vi "decay fit.vi"() -> ()   [LabVIEW 2015]
uses:
  <vilib>/Utility/file.llb/Read Delimited Spreadsheet (DBL).vi
panel:
  out "XY Graph":cluster{"all rows":dbl[], "all rows":dbl[]}[](graph)=[{"all rows"=[5.0, 6.0, 7.0, 8.0, 9.0, 10.0, 11.0, 12.0, 13.0, 14.0, 15.0, 16.0, 17.0, 18.0, 19.0, 20.0, 21.0, 22.0, 23.0, 24.0, 25.0, 26.0, 27.0, 28.0, 29.0, 30.0, 31.0, 32.0, 33.0, 34.0, 35.0, 36.0, 37.0, 38.0, 39.0, 40.0, 41.0, 42.0, 43.0, 44.0, 45.0, 46.0, 47.0, 48.0, 49.0, 50.0, 51.0, 52.0, 53.0, 54.0, 55.0, 56.0, 57.0, 58.0, 59.0, 60.0, 61.0, 62.0, 63.0, 64.0, 65.0, 66.0, 67.0, 68.0, 69.0, 70.0, 71.0, 72.0, 73.0, 74.0, 75.0, 76.0, 77.0, 78.0, 79.0, 80.0, 81.0, 82.0, 83.0, 84.0, 85.0, 86.0, 87.0, 88.0, 89.0, 90.0, 91.0, 92.0, 93.0, 94.0, 95.0, 96.0, 97.0, 98.0, 99.0, 100.0, 101.0, 102.0, 103.0, 104.0, 105.0, 106.0, 107.0, 108.0, 109.0, 110.0, 111.0, 112.0, 113.0, 114.0, 115.0, 116.0, 117.0, 118.0, 119.0, 120.0, 121.0, 122.0, 123.0, 124.0, 125.0, 126.0, 127.0, 128.0, 129.0, 130.0, 131.0, 132.0, 133.0, 134.0, 135.0, 136.0, 137.0, 138.0, 139.0, 140.0, 141.0, 142.0, 143.0, 144.0, 145.0, 146.0, 147.0, 148.0, 149.0, 150.0, 151.0, 152.0, 153.0, 154.0, 155.0, 156.0, 157.0, 158.0, 159.0, 160.0, 161.0, 162.0, 163.0, 164.0, 165.0, 166.0, 167.0, 168.0, 169.0, 170.0, 171.0, 172.0, 173.0, 174.0, 175.0, 176.0, 177.0, 178.0, 179.0, 180.0, 181.0, 182.0, 183.0, 184.0, 185.0, 186.0, 187.0, 188.0, 189.0, 190.0, 191.0, 192.0, 193.0, 194.0, 195.0, 196.0, 197.0, 198.0, 199.0, 200.0, 201.0, 202.0, 203.0, 204.0, 205.0, 206.0, 207.0, 208.0, 209.0, 210.0, 211.0, 212.0, 213.0, 214.0, 215.0, 216.0, 217.0, 218.0, 219.0, 220.0, 221.0, 222.0, 223.0, 224.0, 225.0, 226.0, 227.0, 228.0, 229.0, 230.0, 231.0, 232.0, 233.0, 234.0, 235.0, 236.0, 237.0, 238.0, 239.0, 240.0, 241.0, 242.0, 243.0, 244.0, 245.0, 246.0, 247.0, 248.0, 249.0, 250.0, 251.0, 252.0, 253.0, 254.0, 255.0, 256.0, 257.0, 258.0, 259.0, 260.0, 261.0, 262.0, 263.0, 264.0, 265.0, 266.0, 267.0, 268.0, 269.0, 270.0, 271.0, 272.0, 273.0, 274.0, 275.0, 276.0, 277.0, 278.0, 279.0, 280.0, 281.0, 282.0, 283.0, 284.0, 285.0, 286.0, 287.0, 288.0, 289.0, 290.0, 291.0, 292.0, 293.0, 294.0, 295.0, 296.0, 297.0, 298.0, 299.0], "all rows"=[55.0, 51.0, 55.0, 55.0, 51.0, 65.0, 51.0, 53.0, 44.0, 60.0, 55.0, 45.0, 57.0, 46.0, 54.0, 45.0, 53.0, 58.0, 42.0, 52.0, 57.0, 47.0, 58.0, 46.0, 55.0, 56.0, 43.0, 49.0, 39.0, 47.0, 35.0, 43.0, 32.0, 46.0, 41.0, 43.0, 55.0, 32.0, 54.0, 42.0, 36.0, 36.0, 35.0, 38.0, 39.0, 51.0, 38.0, 53.0, 46.0, 42.0, 37.0, 43.0, 33.0, 35.0, 30.0, 30.0, 37.0, 48.0, 27.0, 32.0, 34.0, 41.0, 34.0, 31.0, 30.0, 39.0, 30.0, 39.0, 28.0, 26.0, 24.0, 23.0, 34.0, 41.0, 17.0, 29.0, 35.0, 31.0, 38.0, 24.0, 29.0, 33.0, 28.0, 38.0, 30.0, 29.0, 28.0, 32.0, 22.0, 23.0, 27.0, 22.0, 34.0, 27.0, 20.0, 20.0, 23.0, 20.0, 27.0, 20.0, 23.0, 23.0, 28.0, 34.0, 20.0, 23.0, 15.0, 19.0, 21.0, 17.0, 22.0, 22.0, 25.0, 21.0, 18.0, 16.0, 17.0, 20.0, 26.0, 27.0, 31.0, 24.0, 18.0, 23.0, 22.0, 16.0, 28.0, 22.0, 21.0, 17.0, 16.0, 20.0, 23.0, 17.0, 11.0, 18.0, 14.0, 20.0, 14.0, 20.0, 20.0, 22.0, 13.0, 14.0, 14.0, 26.0, 18.0, 19.0, 7.0, 21.0, 16.0, 14.0, 19.0, 18.0, 9.0, 12.0, 19.0, 20.0, 20.0, 14.0, 13.0, 11.0, 14.0, 12.0, 14.0, 9.0, 15.0, 10.0, 9.0, 17.0, 11.0, 14.0, 11.0, 12.0, 17.0, 7.0, 20.0, 9.0, 10.0, 9.0, 10.0, 8.0, 17.0, 7.0, 7.0, 10.0, 11.0, 11.0, 17.0, 14.0, 14.0, 11.0, 8.0, 10.0, 7.0, 14.0, 12.0, 12.0, 8.0, 7.0, 9.0, 5.0, 11.0, 10.0, 9.0, 12.0, 10.0, 9.0, 7.0, 11.0, 10.0, 11.0, 10.0, 9.0, 7.0, 8.0, 19.0, 2.0, 5.0, 8.0, 10.0, 8.0, 9.0, 4.0, 10.0, 4.0, 7.0, 10.0, 5.0, 9.0, 9.0, 8.0, 8.0, 5.0, 5.0, 5.0, 7.0, 6.0, 8.0, 12.0, 8.0, 6.0, 10.0, 5.0, 3.0, 5.0, 9.0, 7.0, 9.0, 9.0, 7.0, 12.0, 11.0, 4.0, 7.0, 7.0, 9.0, 3.0, 4.0, 9.0, 7.0, 6.0, 10.0, 5.0, 3.0, 4.0, 6.0, 3.0, 2.0, 6.0, 7.0, 12.0, 9.0, 3.0, 6.0, 6.0, 5.0, 8.0, 9.0, 5.0, 5.0, 6.0, 4.0, 3.0, 8.0, 6.0, 2.0, 8.0, 7.0, 6.0, 6.0, 4.0, 4.0, 5.0, 3.0]}, {"all rows"=[5.0, 6.0, 7.0, 8.0, 9.0, 10.0, 11.0, 12.0, 13.0, 14.0, 15.0, 16.0, 17.0, 18.0, 19.0, 20.0, 21.0, 22.0, 23.0, 24.0, 25.0, 26.0, 27.0, 28.0, 29.0, 30.0, 31.0, 32.0, 33.0, 34.0, 35.0, 36.0, 37.0, 38.0, 39.0, 40.0, 41.0, 42.0, 43.0, 44.0, 45.0, 46.0, 47.0, 48.0, 49.0, 50.0, 51.0, 52.0, 53.0, 54.0, 55.0, 56.0, 57.0, 58.0, 59.0, 60.0, 61.0, 62.0, 63.0, 64.0, 65.0, 66.0, 67.0, 68.0, 69.0, 70.0, 71.0, 72.0, 73.0, 74.0, 75.0, 76.0, 77.0, 78.0, 79.0, 80.0, 81.0, 82.0, 83.0, 84.0, 85.0, 86.0, 87.0, 88.0, 89.0, 90.0, 91.0, 92.0, 93.0, 94.0, 95.0, 96.0, 97.0, 98.0, 99.0, 100.0, 101.0, 102.0, 103.0, 104.0, 105.0, 106.0, 107.0, 108.0, 109.0, 110.0, 111.0, 112.0, 113.0, 114.0, 115.0, 116.0, 117.0, 118.0, 119.0, 120.0, 121.0, 122.0, 123.0, 124.0, 125.0, 126.0, 127.0, 128.0, 129.0, 130.0, 131.0, 132.0, 133.0, 134.0, 135.0, 136.0, 137.0, 138.0, 139.0, 140.0, 141.0, 142.0, 143.0, 144.0, 145.0, 146.0, 147.0, 148.0, 149.0, 150.0, 151.0, 152.0, 153.0, 154.0, 155.0, 156.0, 157.0, 158.0, 159.0, 160.0, 161.0, 162.0, 163.0, 164.0, 165.0, 166.0, 167.0, 168.0, 169.0, 170.0, 171.0, 172.0, 173.0, 174.0, 175.0, 176.0, 177.0, 178.0, 179.0, 180.0, 181.0, 182.0, 183.0, 184.0, 185.0, 186.0, 187.0, 188.0, 189.0, 190.0, 191.0, 192.0, 193.0, 194.0, 195.0, 196.0, 197.0, 198.0, 199.0, 200.0, 201.0, 202.0, 203.0, 204.0, 205.0, 206.0, 207.0, 208.0, 209.0, 210.0, 211.0, 212.0, 213.0, 214.0, 215.0, 216.0, 217.0, 218.0, 219.0, 220.0, 221.0, 222.0, 223.0, 224.0, 225.0, 226.0, 227.0, 228.0, 229.0, 230.0, 231.0, 232.0, 233.0, 234.0, 235.0, 236.0, 237.0, 238.0, 239.0, 240.0, 241.0, 242.0, 243.0, 244.0, 245.0, 246.0, 247.0, 248.0, 249.0, 250.0, 251.0, 252.0, 253.0, 254.0, 255.0, 256.0, 257.0, 258.0, 259.0, 260.0, 261.0, 262.0, 263.0, 264.0, 265.0, 266.0, 267.0, 268.0, 269.0, 270.0, 271.0, 272.0, 273.0, 274.0, 275.0, 276.0, 277.0, 278.0, 279.0, 280.0, 281.0, 282.0, 283.0, 284.0, 285.0, 286.0, 287.0, 288.0, 289.0, 290.0, 291.0, 292.0, 293.0, 294.0, 295.0, 296.0, 297.0, 298.0, 299.0], "all rows"=[57.869919492504515, 57.37134834923303, 56.87707258406269, 56.387055190694035, 55.90125948165079, 55.41964908553312, 54.942187944294496, 54.468840310542014, 53.99957074486004, 53.53434411315681, 53.07312558403405, 52.61588062617905, 52.16257500577936, 51.71317478395972, 51.26764631424108, 50.82595624002143, 50.38807149207849, 49.95395928609374, 49.52358712019794, 49.09692277253767, 48.6739342988629, 48.254590030135375, 47.8388585701575, 47.426708793221735, 47.01810984178026, 46.61303112413461, 46.21144231214535, 45.81331333896137, 45.4186143967688, 45.02731593455932, 44.63938865591765, 44.25480351682819, 43.87353172350043, 43.49554473021324, 43.12081423717762, 42.749312188417875, 42.381010769671136, 42.01588240630486, 41.65389976125237, 41.295035732966085, 40.93926345338846, 40.586556285940404, 40.23688782352696, 39.89023188656026, 39.546562520999395, 39.20585399640735, 38.868080804024466, 38.533217654858674, 38.20123947779209, 37.87212141770394, 37.54583883360968, 37.222367296816124, 36.90168258909248, 36.58376070085712, 36.268577829380014, 35.9561103770006, 35.64633494936105, 35.33922835365475, 35.03476759688981, 34.73292988416767, 34.43369261697636, 34.13703339149864, 33.842929996934544, 33.55136041383855, 33.26230281247093, 32.97573555116337, 32.6916371746987, 32.40998641270451, 32.13076217806067, 31.85394356532051, 31.579509849145666, 31.30744048275436, 31.037715096383078, 30.77031349576148, 30.5052156606005, 30.24240174309334, 29.981852066429585, 29.72354712332193, 29.46746757454568, 29.213594247490857, 28.961908134726745, 28.712390392578776, 28.46502233971775, 28.219785455761148, 27.97666137988651, 27.735631909456785, 27.496678998657487, 27.25978475714562, 27.024931448710227, 26.792101489944482, 26.56127744892923, 26.332442043927863, 26.10557814209244, 25.880668758180963, 25.657697053285677, 25.436646333572355, 25.217500049030452, 25.000241792233975, 24.7848552971131, 24.571324437736315, 24.35963322710307, 24.149765815946854, 23.94170649154854, 23.73543967656001, 23.53094992783785, 23.328221935287146, 23.12724052071522, 22.927990636695235, 22.730457365439594, 22.534625917683062, 22.340481631575503, 22.148009971584116, 21.95719652740521, 21.76802701288527, 21.58048726495138, 21.39456324255083, 21.21024102559986, 21.027506813941475, 20.846346926312226, 20.666747799317907, 20.488695986418044, 20.31217815691919, 20.13718109497683, 19.963691698605924, 19.79169697869997, 19.62118405805851, 19.45214017042301, 19.28455265952106, 19.11840897811881, 18.953696687081546, 18.790403454442384, 18.628517054478976, 18.46802536679818, 18.308916375428595, 18.15117816792095, 17.9947989344562, 17.83976696696134, 17.686070658232815, 17.533698501067512, 17.382639087401195, 17.2328811074544, 17.08441334888567, 16.937224695952086, 16.79130412867705, 16.646640722025207, 16.503223645084486, 16.361042160255213, 16.220085622446174, 16.080343478277616, 15.941805265291139, 15.804460611166345, 15.668299232944301, 15.533310936257614, 15.399485614567226, 15.266813248405699, 15.135283904627094, 15.004887735663255, 14.875614978786535, 14.747455955378863, 14.620401070207103, 14.49444081070467, 14.369565746259319, 14.245766527507076, 14.123033885632262, 14.001358631673535, 13.880731655835913, 13.761143926808725, 13.642586491089446, 13.525050472313344, 13.408527070588908, 13.293007561839014, 13.178483297147736, 13.064945702112821, 12.95238627620372, 12.840796592125152, 12.730168295186159, 12.62049310267459, 12.511762803236982, 12.403969256263766, 12.297104391279795, 12.191160207340102, 12.086128772430872, 11.982002222875577, 11.87877276274622, 11.776432663279664, 11.67497426229897, 11.574389963639742, 11.4746722365814, 11.375813615283354, 11.277806698226044, 11.180644147656785, 11.084318689040398, 10.988823110514561, 10.894150262349863, 10.800293056414494, 10.707244465643582, 10.61499752351306, 10.52354532351808, 10.432881018655944, 10.342997820913455, 10.25388900075871, 10.165547886637246, 10.077967864472566, 9.991142377170927, 9.905064924130414, 9.819729060754252, 9.735128397968285, 9.65125660174264, 9.5681073926175, 9.485674545232953, 9.40395188786291, 9.32293330195302, 9.242612721662589, 9.162984133410419, 9.08404157542458, 9.00577913729605, 8.92819095953621, 8.851271233138133, 8.775014199141685, 8.699414148202333, 8.624465420163698, 8.550162403633783, 8.476499535564844, 8.403471300836884, 8.331072231844745, 8.259296908088746, 8.188139955768849, 8.117596047382328, 8.047659901324897, 7.978326281495285, 7.909589996903197, 7.841445901280677, 7.773888892696808, 7.706913913175723, 7.640515948317925, 7.574690026924856, 7.509431220626702, 7.444734643513417, 7.3805954517689045, 7.317008843308367, 7.253970057418776, 7.191474374402441, 7.129517115223641, 7.06809364115831, 7.007199353446737, 6.946829692949253, 6.886980139804902, 6.827646213093024, 6.768823470497781, 6.710507507975559, 6.6526939594252354, 6.595378496361293, 6.538556827589749, 6.4822246988868715, 6.426377892680665, 6.371012227735108, 6.3161235588370985, 6.26170777648611, 6.207760806586506, 6.154278610142521, 6.101257182955856, 6.04869255532589, 5.996580791752464, 5.9449179906412395, 5.893700284011579, 5.842923837206953, 5.792584848607846, 5.7426795493471205, 5.693204203027853, 5.644155105443585, 5.595528584300989, 5.5473209989449295, 5.499528740085885, 5.452148229529721, 5.405175919909792, 5.358608294421356, 5.312441866558263, 5.266673179851928, 5.221298807612545, 5.176315352672529, 5.131719447132175, 5.087507752107498, 5.04367695748026, 5.000223781650136, 4.95714497128902, 4.91443730109746, 4.872097573563166, 4.830122618721623, 4.788509293918754, 4.747254483575628, 4.706355098955203, 4.665808077931067, 4.625610384758179, 4.585759009845587, 4.546250969531095]}]
  in  "file path (dialog if empty)":path
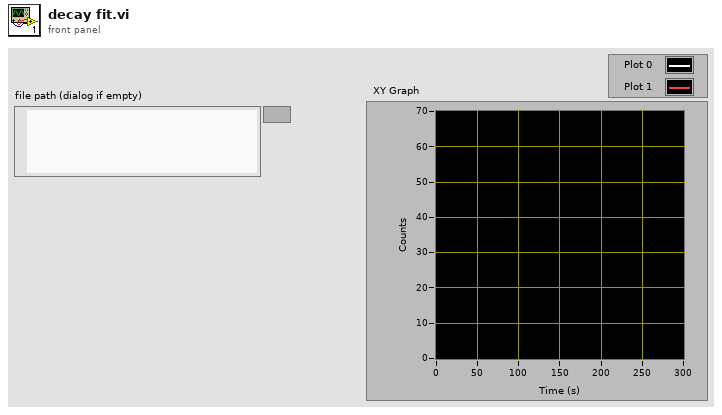
[diagram p1: front panel]
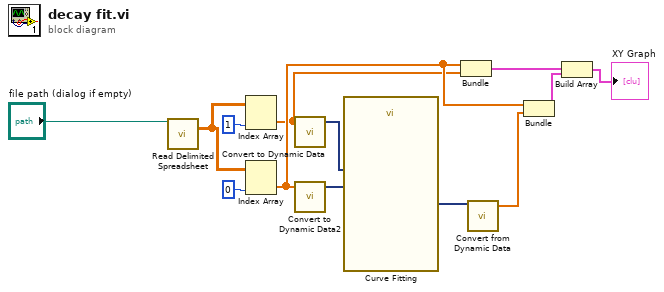
[diagram p0: block diagram]
diagram:
  n1 = call-poly <vilib>:"Read Delimited Spreadsheet.vi"("file path (dialog if empty)"="file path (dialog if empty)") -> ("all rows"=w8:dbl[][])  [unwired: 9 in, 5 out]
  n2 = Index Array(array=w8, index (col)=1 ("disabled index (col)")) -> (element=w4:dbl[])  [unwired: 1 in]
  n3 = Index Array(array=w8, index (col)=0 ("disabled index (col)")) -> (element=w5:dbl[])  [unwired: 1 in]
  n4 = call "Convert to Dynamic Data"("Array"=w4) -> ("Dynamic Data Type"=w10:dynamicdata)  [unwired: 3 in]
  n5 = call "Convert to Dynamic Data2"("Array"=w5) -> ("Dynamic Data Type"=w11:dynamicdata)  [unwired: 3 in]
  n6 = call "Curve Fitting"("Locations"=w11, "Signals"=w10) -> ("best fit"=w7:dynamicdata)  [unwired: 5 in, 4 out]
  n7 = Bundle("all rows"=w5, "all rows"=w4) -> (w2:cluster{"all rows":dbl[], "all rows":dbl[]})  [unwired: 1 in]
  n8 = call "Convert from Dynamic Data"("Dynamic Data Type"=w7) -> ("Array"=w6:dbl[])  [unwired: 3 in]
  n9 = Bundle("all rows"=w5, "Array"=w6) -> (w1:cluster{"all rows":dbl[], "Array":dbl[]})  [unwired: 1 in]
  n10 = Build Array(w2, w1) -> (→"XY Graph":cluster{"all rows":dbl[], "Array":dbl[]}[])
